vi "NF LI56xx dvr psd1Y OFFSet.vi"(8 "error in":errorcluster caption="error in (no error)" {"code" format="%.0x"}, 9 "Read(F)":bool, 10 "set offset value":dbl min=-105.0 max=105.0 step=0.001 format="%#.3f", 11 "VISA resource name":refnum<visa-resource-name>) -> (0 "error out":errorcluster {"code" format="%.0x"}, 2 "query offset value":string, 3 "VISA resource name copy":refnum<visa-resource-name>)   [LabVIEW 2019]
doc: "Sets/queries the offset for the primary PSD's Y output. \nFor offset adjustment, also enable offset with the \n:CALCulate2:OFFSet:STATe ON command."
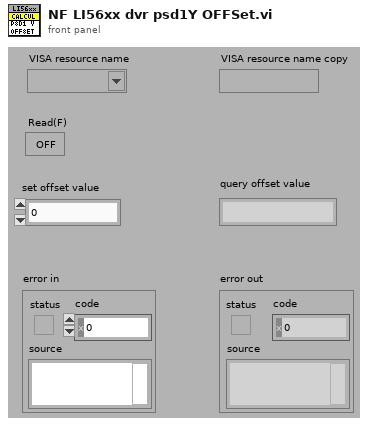
[diagram p1: front panel]
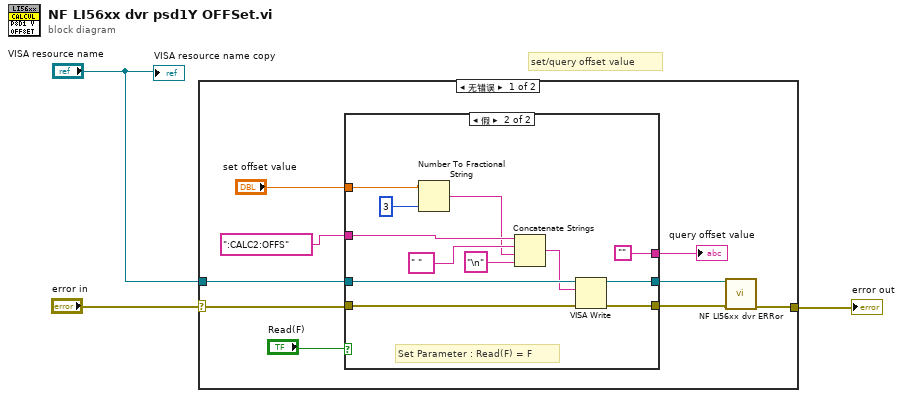
[diagram p0: block diagram]
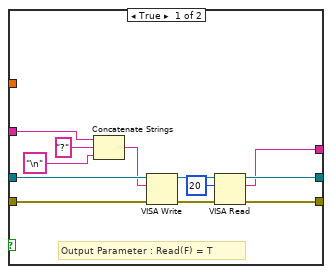
[diagram p2: hidden frame]
diagram:
  # "set/query offset value"
  n1 = case shown="无错误" "error in" {
    selector: "error in" -> [w11 w37]
    tunnel: [w5 w37] -> w3
    tunnel: "VISA resource name" -> [w10 _]
    frame No Error {
      n2 = case shown="假" "Read(F)" {
        tunnel: w10 -> [w24 w36]
        tunnel: [w21 w33] -> w7
        tunnel: [w20 w34] -> w6
        tunnel: w11 -> [w19 w35]
        tunnel: [w15 ""] -> w9
        tunnel: "set offset value" -> [_ w27]
        tunnel: ":CALC2:OFFS" ("•¶Žš—ñ") -> [w13 w28]
        frame True {
          # "Output Parameter : Read(F) = T"
          n3 = Concatenate Strings(w13, "?" ("Œ`Ž®•¶Žš—ñ"), "\n" ("Œ`Ž®•¶Žš—ñ")) -> (w16:string)
          n4 = VISA Write(VISA resource name=w24, write buffer=w16, error in (no error)=w19) -> (VISA resource name out=w22:refnum<visa-resource-name>, error out=w23:errorcluster)  [unwired: 1 out]
          n5 = VISA Read(VISA resource name=w22, byte count=u32 20 ("バイトカウント（0）"), error in (no error)=w23) -> (VISA resource name out=w21:refnum<visa-resource-name>, read buffer=w15:string, error out=w20:errorcluster)  [unwired: 1 out]
        }
        frame False {
          # "Set Parameter : Read(F) = F"
          n6 = Number To Fractional String(number=w27, precision (6)=i16 3 ("¸x (6)")) -> (F-format string=w25:string)  [unwired: 2 in]
          n7 = Concatenate Strings(w28, " ", w25, "\n" ("Œ`Ž®•¶Žš—ñ")) -> (w31:string)
          n8 = VISA Write(VISA resource name=w36, write buffer=w31, error in (no error)=w35) -> (VISA resource name out=w33:refnum<visa-resource-name>, error out=w34:errorcluster)  [unwired: 1 out]
        }
      }
      "query offset value" <- w9
      n9 = call "NF LI56xx dvr ERRor.vi"("VISA resource name"=w7, "error in (no error)"=w6) -> ("error out"=w5:errorcluster)  [unwired: 10 in, 3 out]
    }
    frame Error {
    }
  }
  "error out" <- w3
  "VISA resource name copy" <- "VISA resource name"
